vi "getDetails.vi"(8 "error in (no error)":errorcluster, 9 "S/N":string, 10 "Device Type":T1=enum."k4b2", 11 "reference in":refnum<class "Devices Controller.lvclass">) -> (0 "error out":errorcluster, 2 "details":T2, 3 "reference out":refnum<class "Devices Controller.lvclass">)   [LabVIEW 2014, in "Devices Controller.lvclass"]
uses:
  Devices Controller.lvclass
  deviceType.ctl
  APP/k4b2_class/k4b2.lvclass
  APP/fitmate_class/fitmate.lvclass
  APP/cpet_class/cpet.lvclass
  APP/rmr_class/rmr.lvclass
  APP/bodpod_class/bodpod.lvclass
  APP/peapod_class/peapod.lvclass
  APP/bb-pft_class/bb-pft.lvclass
  APP/k5_class/k5.lvclass
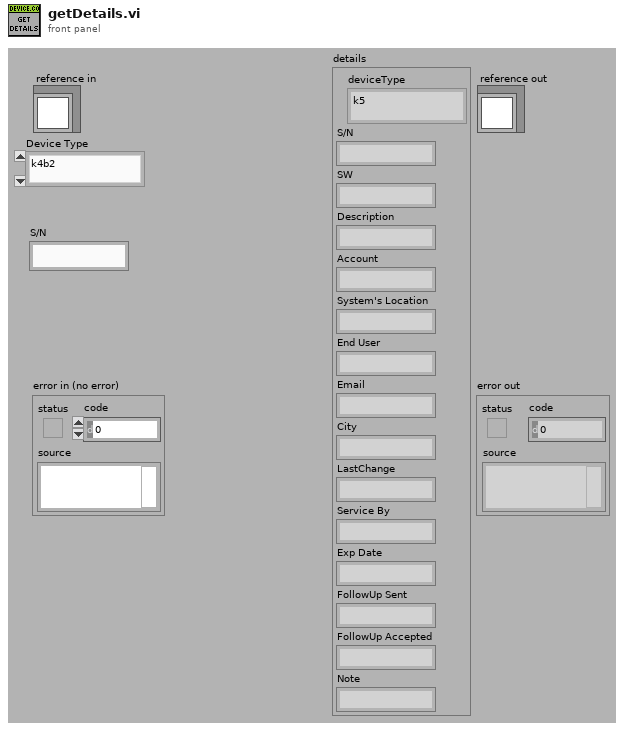
[diagram p1: front panel]
types:
  T1 = typedef "Devices Controller.lvclass/deviceType.ctl" = enum16{"k5", "k4b2", "fitmate", "cpet", "rmr", "bodyBoxPft", "bp", "pp"}
  T2 = cluster{"deviceType":T1, "S/N":string, "SW":string, "Description":string, "Account":string, "System's Location":string, "End User":string, "Email":string, "City":string, "LastChange":string, "Service By":string, "Exp Date":string, "FollowUp Sent":string, "FollowUp Accepted":string, "Note":string}
  T3 = typedef "Devices Controller.lvclass/ObjectAttributesRef.ctl" = refnum<data-value>
  T4 = typedef "Devices Controller.lvclass/ObjectAttributes.ctl" = cluster{"MyAttribute":dbl, "file_controller_ref":refnum<class "File Controller.lvclass">, "data":string[][][], "devices_refs":cluster{"k4b2_refs":refnum<class "k4b2.lvclass">[], "rmr_refs":refnum<class "rmr.lvclass">[], "bod_pod_refs":refnum<class "bodpod.lvclass">[], "cpet_refs":refnum<class "cpet.lvclass">[], "fitmate_refs":refnum<class "fitmate.lvclass">[], "pea_pod_refs":refnum<class "peapod.lvclass">[], "k5_refs":refnum<class "k5.lvclass">[], "bb-pft_refs":refnum<class "bb-pft.lvclass">[]}}
  T5 = cluster{"k4b2_refs":refnum<class "k4b2.lvclass">[], "rmr_refs":refnum<class "rmr.lvclass">[], "bod_pod_refs":refnum<class "bodpod.lvclass">[], "cpet_refs":refnum<class "cpet.lvclass">[], "fitmate_refs":refnum<class "fitmate.lvclass">[], "pea_pod_refs":refnum<class "peapod.lvclass">[], "k5_refs":refnum<class "k5.lvclass">[], "bb-pft_refs":refnum<class "bb-pft.lvclass">[]}
  T6 = cluster{"deviceType":T1, "S/N":string, "SW":string, "Description":string, "Account":string, "System's Location":string, "End User":string, "Email":string, "City":string, "FollowUp Sent":string, "FollowUp Accepted":string, "Note":string}
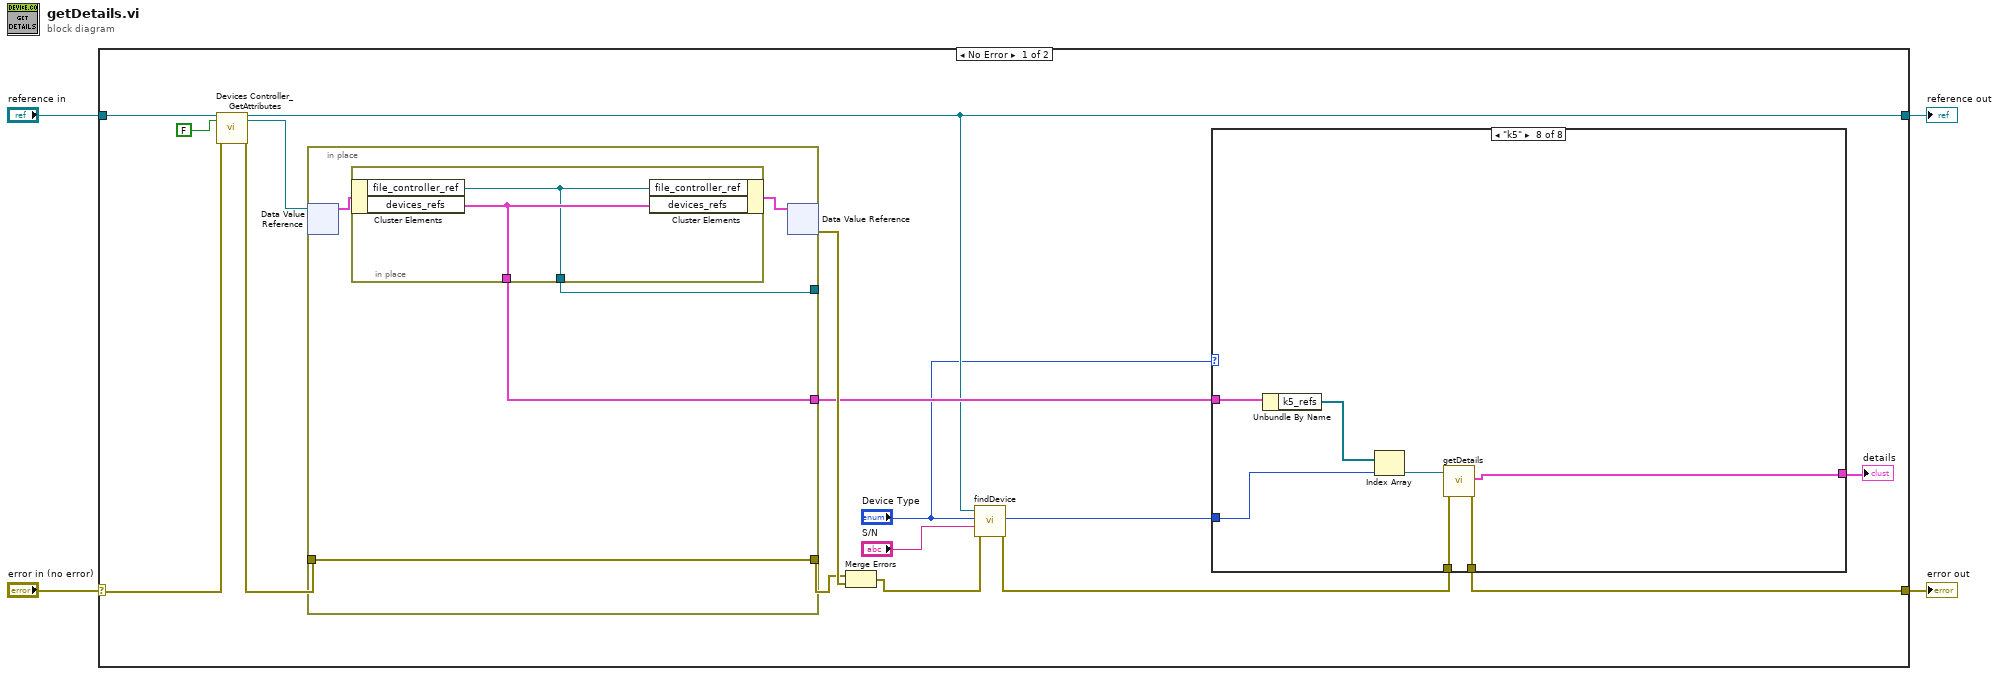
[diagram p0: block diagram]
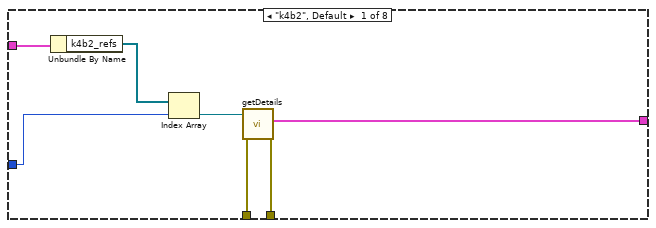
[diagram p2: hidden frame]
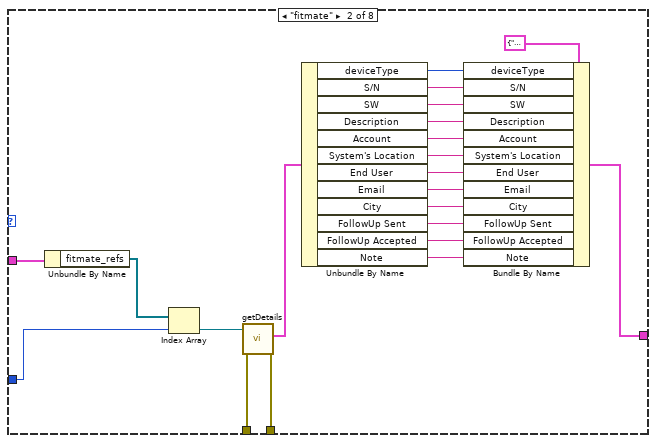
[diagram p3: hidden frame]
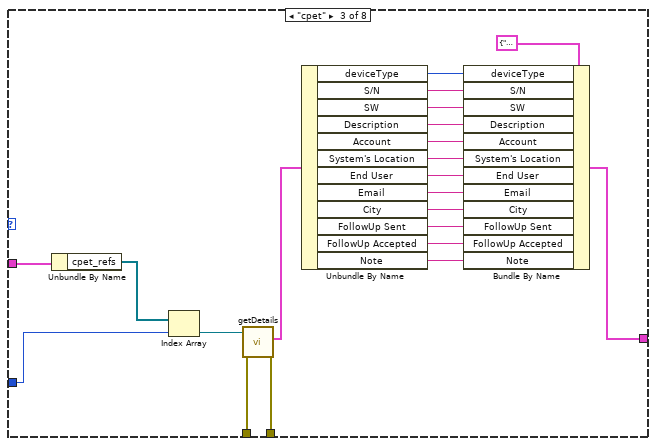
[diagram p4: hidden frame]
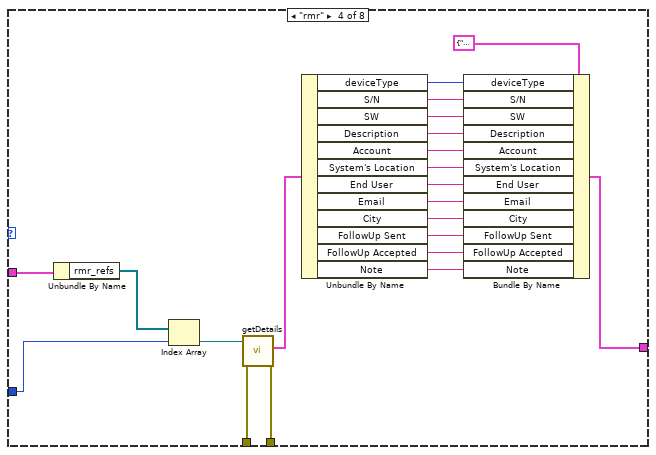
[diagram p5: hidden frame]
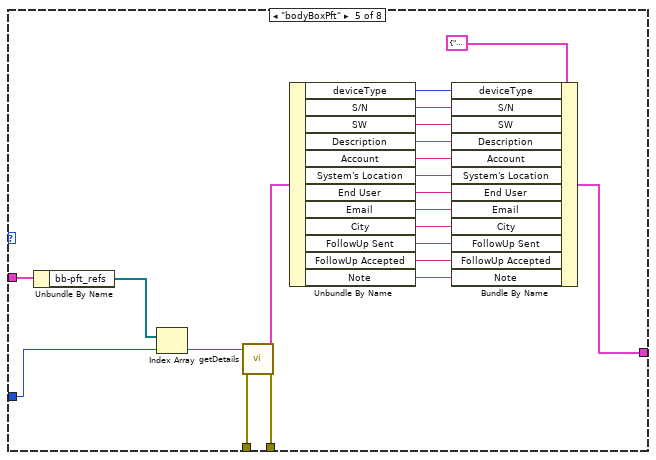
[diagram p6: hidden frame]
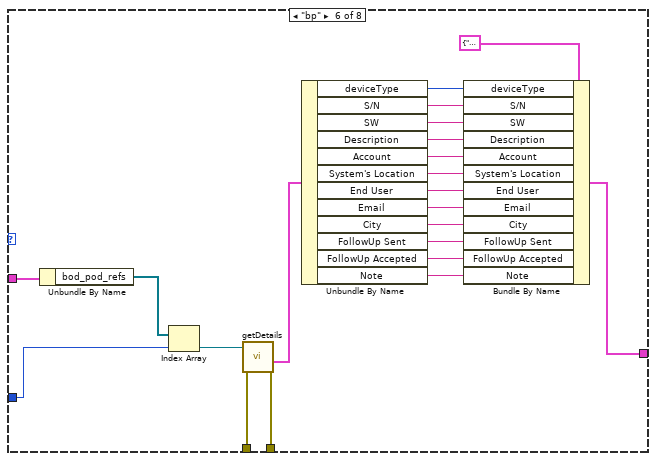
[diagram p7: hidden frame]
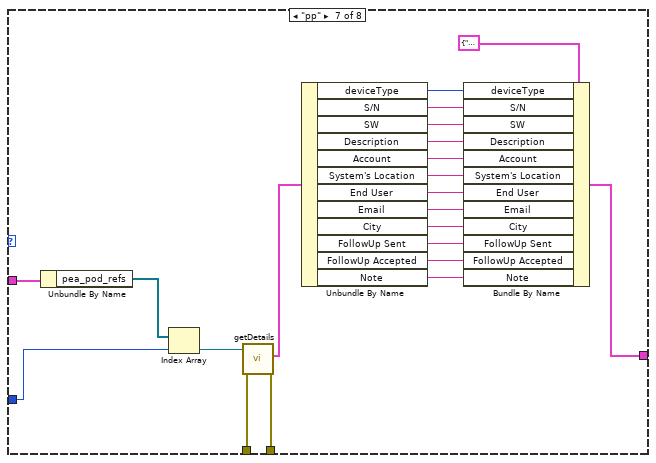
[diagram p8: hidden frame]
diagram:
  n1 = case shown="No Error" "error in (no error)" {
    selector: "error in (no error)" -> [w16 w169]
    tunnel: [w12 w169] -> w3
    tunnel: [w11 w168] -> w1
    tunnel: "reference in" -> [w18 w168]
    frame No Error {
      n2 = call "Devices Controller_GetAttributes.vi"("reference in"=w18, "return data? (T)"=FALSE, "error in (no error)"=w16) -> ("reference out"=w11:refnum<class "Devices Controller.lvclass">, "attributes ref"=w14:T3, "error out"=w15:errorcluster)  [unwired: 13 in, 1 out]
      n3 = in-place {
        in-place-border: w15 -> [w163]
        in-place-border: [w163] -> w19
        in-place-border: [w162] -> w13
        in-place-border: [w161] -> _
        n4 = in-place-dvr #1(w14) -> (w164:T4)  [unwired: 1 out]
        n5 = in-place {
          in-place-border: [w167] -> w162
          in-place-border: [w166] -> w161
          n6 = in-place-cluster #2(w164) -> ("file_controller_ref"=w166:refnum<class "File Controller.lvclass">, "devices_refs"=w167:T5)
          n7 = in-place-cluster #2("file_controller_ref"=w166, "devices_refs"=w167) -> (w165:T4)
        }
        n8 = in-place-dvr #1(w165) -> (w20:errorcluster)  [unwired: 1 out]
      }
      n9 = Merge Errors(w19, w20) -> (w9:errorcluster)
      n10 = call "findDevice.vi"("error in (no error)"=w9, "S/N:"="S/N", "Device Type:"="Device Type", "reference in"=w11) -> ("error out"=w8:errorcluster, "index of element"=w7:i32)  [unwired: 4 in, 2 out]
      n11 = case shown="\"k5\"" "Device Type" {
        tunnel: w13 -> [w27 w48 w69 w90 w91 w132 w153 w158]
        tunnel: w7 -> [w22 w44 w65 w86 w95 w128 w149 w154]
        tunnel: w8 -> [w26 w47 w68 w89 w94 w131 w152 w157]
        tunnel: [w25 w46 w67 w88 w93 w130 w151 w156] -> w12
        tunnel: [w24 w29 w49 w70 w92 w112 w133 w155] -> w5
        frame "k4b2", Default {
          n12 = Unbundle By Name(w27) -> ("k4b2_refs"=w23:refnum<class "k4b2.lvclass">[])
          n13 = Index Array(array=w23, index=w22) -> (element=w21:refnum<class "k4b2.lvclass">)
          n14 = call "getDetails.vi"("error in (no error)"=w26, "reference in"=w21) -> ("error out"=w25:errorcluster, "details"=w24:T2)  [unwired: 7 in, 1 out]
        }
        frame "fitmate" {
          n15 = Unbundle By Name(w48) -> ("fitmate_refs"=w45:refnum<class "fitmate.lvclass">[])
          n16 = Index Array(array=w45, index=w44) -> (element=w43:refnum<class "fitmate.lvclass">)
          n17 = call "getDetails.vi"("error in (no error)"=w47, "reference in"=w43) -> ("error out"=w46:errorcluster, "details"=w42:T6)  [unwired: 7 in, 1 out]
          n18 = Unbundle By Name(w42) -> ("deviceType"=w41:T1, "S/N"=w40:string, "SW"=w39:string, "Description"=w38:string, "Account"=w37:string, "System's Location"=w36:string, "End User"=w35:string, "Email"=w34:string, "City"=w33:string, "FollowUp Sent"=w32:string, "FollowUp Accepted"=w31:string, "Note"=w28:string)
          n19 = Bundle By Name(cluster=T2 {"deviceType"=enum."k5", "S/N"="", "SW"="", "Description"="", "Account"="", "System's Location"="", "End User"="", "Email"="", "City"="", "LastChange"="", "Service By"="", "Exp Date"="", "FollowUp Sent"="", "FollowUp Accepted"="", "Note"=""} ("details"), "deviceType"=w41, "S/N"=w40, "SW"=w39, "Description"=w38, "Account"=w37, "System's Location"=w36, "End User"=w35, "Email"=w34, "City"=w33, "FollowUp Sent"=w32, "FollowUp Accepted"=w31, "Note"=w28) -> (w29:T2)
        }
        frame "cpet" {
          n20 = Unbundle By Name(w69) -> ("cpet_refs"=w66:refnum<class "cpet.lvclass">[])
          n21 = Index Array(array=w66, index=w65) -> (element=w64:refnum<class "cpet.lvclass">)
          n22 = call "getDetails.vi"("error in (no error)"=w68, "reference in"=w64) -> ("error out"=w67:errorcluster, "details"=w63:T6)  [unwired: 7 in, 1 out]
          n23 = Unbundle By Name(w63) -> ("deviceType"=w62:T1, "S/N"=w61:string, "SW"=w60:string, "Description"=w59:string, "Account"=w58:string, "System's Location"=w57:string, "End User"=w56:string, "Email"=w55:string, "City"=w54:string, "FollowUp Sent"=w53:string, "FollowUp Accepted"=w52:string, "Note"=w50:string)
          n24 = Bundle By Name(cluster=T2 {"deviceType"=enum."k5", "S/N"="", "SW"="", "Description"="", "Account"="", "System's Location"="", "End User"="", "Email"="", "City"="", "LastChange"="", "Service By"="", "Exp Date"="", "FollowUp Sent"="", "FollowUp Accepted"="", "Note"=""} ("details"), "deviceType"=w62, "S/N"=w61, "SW"=w60, "Description"=w59, "Account"=w58, "System's Location"=w57, "End User"=w56, "Email"=w55, "City"=w54, "FollowUp Sent"=w53, "FollowUp Accepted"=w52, "Note"=w50) -> (w49:T2)
        }
        frame "rmr" {
          n25 = Unbundle By Name(w90) -> ("rmr_refs"=w87:refnum<class "rmr.lvclass">[])
          n26 = Index Array(array=w87, index=w86) -> (element=w85:refnum<class "rmr.lvclass">)
          n27 = call "getDetails.vi"("error in (no error)"=w89, "reference in"=w85) -> ("error out"=w88:errorcluster, "details"=w84:T6)  [unwired: 7 in, 1 out]
          n28 = Unbundle By Name(w84) -> ("deviceType"=w83:T1, "S/N"=w82:string, "SW"=w81:string, "Description"=w80:string, "Account"=w79:string, "System's Location"=w78:string, "End User"=w77:string, "Email"=w76:string, "City"=w75:string, "FollowUp Sent"=w74:string, "FollowUp Accepted"=w73:string, "Note"=w72:string)
          n29 = Bundle By Name(cluster=T2 {"deviceType"=enum."k5", "S/N"="", "SW"="", "Description"="", "Account"="", "System's Location"="", "End User"="", "Email"="", "City"="", "LastChange"="", "Service By"="", "Exp Date"="", "FollowUp Sent"="", "FollowUp Accepted"="", "Note"=""} ("details"), "deviceType"=w83, "S/N"=w82, "SW"=w81, "Description"=w80, "Account"=w79, "System's Location"=w78, "End User"=w77, "Email"=w76, "City"=w75, "FollowUp Sent"=w74, "FollowUp Accepted"=w73, "Note"=w72) -> (w70:T2)
        }
        frame "bodyBoxPft" {
          n30 = Unbundle By Name(w91) -> ("bb-pft_refs"=w111:refnum<class "bb-pft.lvclass">[])
          n31 = Index Array(array=w111, index=w95) -> (element=w110:refnum<class "bb-pft.lvclass">)
          n32 = call "getDetails.vi"("error in (no error)"=w94, "reference in"=w110) -> ("error out"=w93:errorcluster, "details"=w109:T6)  [unwired: 7 in, 1 out]
          n33 = Unbundle By Name(w109) -> ("deviceType"=w108:T1, "S/N"=w107:string, "SW"=w106:string, "Description"=w105:string, "Account"=w104:string, "System's Location"=w103:string, "End User"=w102:string, "Email"=w101:string, "City"=w100:string, "FollowUp Sent"=w99:string, "FollowUp Accepted"=w98:string, "Note"=w96:string)
          n34 = Bundle By Name(cluster=T2 {"deviceType"=enum."k5", "S/N"="", "SW"="", "Description"="", "Account"="", "System's Location"="", "End User"="", "Email"="", "City"="", "LastChange"="", "Service By"="", "Exp Date"="", "FollowUp Sent"="", "FollowUp Accepted"="", "Note"=""} ("details"), "deviceType"=w108, "S/N"=w107, "SW"=w106, "Description"=w105, "Account"=w104, "System's Location"=w103, "End User"=w102, "Email"=w101, "City"=w100, "FollowUp Sent"=w99, "FollowUp Accepted"=w98, "Note"=w96) -> (w92:T2)
        }
        frame "bp" {
          n35 = Unbundle By Name(w132) -> ("bod_pod_refs"=w129:refnum<class "bodpod.lvclass">[])
          n36 = Index Array(array=w129, index=w128) -> (element=w127:refnum<class "bodpod.lvclass">)
          n37 = call "getDetails.vi"("error in (no error)"=w131, "reference in"=w127) -> ("error out"=w130:errorcluster, "details"=w126:T6)  [unwired: 7 in, 1 out]
          n38 = Unbundle By Name(w126) -> ("deviceType"=w125:T1, "S/N"=w124:string, "SW"=w123:string, "Description"=w122:string, "Account"=w121:string, "System's Location"=w120:string, "End User"=w119:string, "Email"=w118:string, "City"=w117:string, "FollowUp Sent"=w116:string, "FollowUp Accepted"=w115:string, "Note"=w113:string)
          n39 = Bundle By Name(cluster=T2 {"deviceType"=enum."k5", "S/N"="", "SW"="", "Description"="", "Account"="", "System's Location"="", "End User"="", "Email"="", "City"="", "LastChange"="", "Service By"="", "Exp Date"="", "FollowUp Sent"="", "FollowUp Accepted"="", "Note"=""} ("details"), "deviceType"=w125, "S/N"=w124, "SW"=w123, "Description"=w122, "Account"=w121, "System's Location"=w120, "End User"=w119, "Email"=w118, "City"=w117, "FollowUp Sent"=w116, "FollowUp Accepted"=w115, "Note"=w113) -> (w112:T2)
        }
        frame "pp" {
          n40 = Unbundle By Name(w153) -> ("pea_pod_refs"=w150:refnum<class "peapod.lvclass">[])
          n41 = Index Array(array=w150, index=w149) -> (element=w148:refnum<class "peapod.lvclass">)
          n42 = call "getDetails.vi"("error in (no error)"=w152, "reference in"=w148) -> ("error out"=w151:errorcluster, "details"=w147:T6)  [unwired: 7 in, 1 out]
          n43 = Unbundle By Name(w147) -> ("deviceType"=w146:T1, "S/N"=w145:string, "SW"=w144:string, "Description"=w143:string, "Account"=w142:string, "System's Location"=w141:string, "End User"=w140:string, "Email"=w139:string, "City"=w138:string, "FollowUp Sent"=w137:string, "FollowUp Accepted"=w136:string, "Note"=w134:string)
          n44 = Bundle By Name(cluster=T2 {"deviceType"=enum."k5", "S/N"="", "SW"="", "Description"="", "Account"="", "System's Location"="", "End User"="", "Email"="", "City"="", "LastChange"="", "Service By"="", "Exp Date"="", "FollowUp Sent"="", "FollowUp Accepted"="", "Note"=""} ("details"), "deviceType"=w146, "S/N"=w145, "SW"=w144, "Description"=w143, "Account"=w142, "System's Location"=w141, "End User"=w140, "Email"=w139, "City"=w138, "FollowUp Sent"=w137, "FollowUp Accepted"=w136, "Note"=w134) -> (w133:T2)
        }
        frame "k5" {
          n45 = Unbundle By Name(w158) -> ("k5_refs"=w160:refnum<class "k5.lvclass">[])
          n46 = Index Array(array=w160, index=w154) -> (element=w159:refnum<class "k5.lvclass">)
          n47 = call "getDetails.vi"("error in (no error)"=w157, "reference in"=w159) -> ("error out"=w156:errorcluster, "details"=w155:T2)  [unwired: 7 in, 1 out]
        }
      }
      "details" <- w5
    }
    frame Error {
    }
  }
  "error out" <- w3
  "reference out" <- w1
